vi "Set Get Model.vi"(8 "Error In":errorcluster, 10 "Action":enum16{"Set Model", "Get Model"}(ring), 11 "Model":enum16{"Estar Centauro", "GFL"}(ring)) -> (0 "Error Out":errorcluster, 3 "Model Out":enum16{"Estar Centauro", "GFL"}(ring))   [LabVIEW 2023]
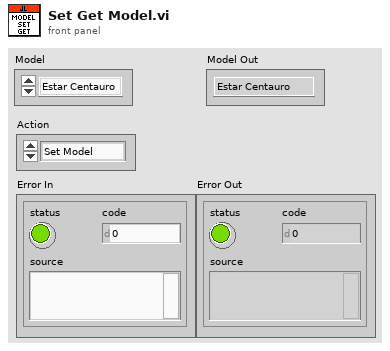
[diagram p1: front panel]
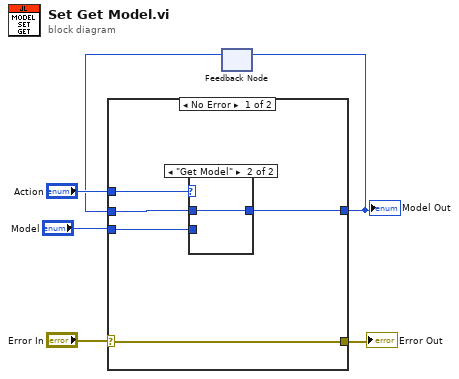
[diagram p0: block diagram]
diagram:
  n1 = feedback #1() -> (w1:enum16{"Estar Centauro", "GFL"})  [unwired: 1 in]
  n2 = case shown="No Error" "Error In" {
    selector: "Error In" -> [w8 w15]
    tunnel: "Action" -> [w11 _]
    tunnel: "Model" -> [w10 _]
    tunnel: [w9 w14] -> w2
    tunnel: [w8 w15] -> w4
    tunnel: w1 -> [w7 w14]
    frame No Error {
      n3 = case shown="\"Get Model\"" w11 {
        tunnel: w10 -> [w12 _]
        tunnel: [w12 w13] -> w9
        tunnel: w7 -> [_ w13]
        frame "Set Model" {
        }
        frame "Get Model" {
        }
      }
    }
    frame Error {
    }
  }
  "Error Out" <- w4
  "Model Out" <- w2
  n4 = feedback-in #1(w2) -> ()
